vi "OF2 (SubVI).vi"() -> (0 "error out":errorcluster, 1 "Optical Flow Velocity X":T1, 2 "Optical Flow Previous Image":T1, 3 "Optical Flow Velocity Y":T1, 5 "Optical Flow Current Image":T1)   [LabVIEW 2014]
uses:
  <vilib>/vision/Image Controls.llb/IMAQ Image.ctl
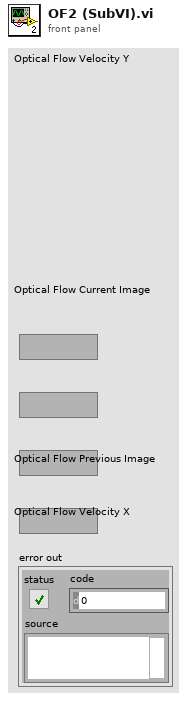
[diagram p1: front panel]
types:
  T1 = typedef "IMAQ Image.ctl" = refnum<image>
  T2 = typedef "Image Type" = u32
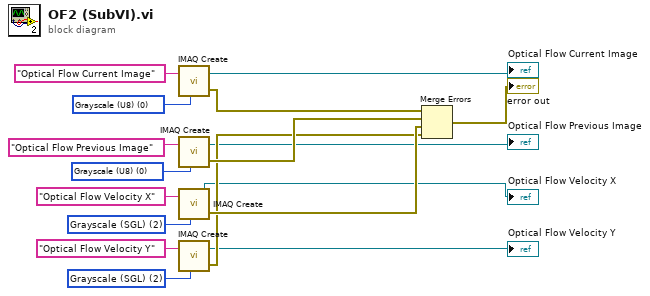
[diagram p0: block diagram]
diagram:
  w8 = T2 2 items=["Grayscale (U8)", "Grayscale (I16)", "Grayscale (SGL)", "Complex (CSG)", "RGB (U32)", "HSL (U32)", "RGB (U64)", "Grayscale (U16)"] ("Image Type")
  w7 = T2 0 items=["Grayscale (U8)", "Grayscale (I16)", "Grayscale (SGL)", "Complex (CSG)", "RGB (U32)", "HSL (U32)", "RGB (U64)", "Grayscale (U16)"] ("Image Type")
  w6 = T2 0 items=["Grayscale (U8)", "Grayscale (I16)", "Grayscale (SGL)", "Complex (CSG)", "RGB (U32)", "HSL (U32)", "RGB (U64)", "Grayscale (U16)"] ("Image Type")
  w5 = T2 2 items=["Grayscale (U8)", "Grayscale (I16)", "Grayscale (SGL)", "Complex (CSG)", "RGB (U32)", "HSL (U32)", "RGB (U64)", "Grayscale (U16)"] ("Image Type")
  n1 = call "IMAQ Create"("Image Name"="Optical Flow Current Image", "Image Type"=w6) -> ("New Image"=→"Optical Flow Current Image":T1, "error out"=w16:errorcluster)  [unwired: 2 in, 1 out]
  n2 = call "IMAQ Create"("Image Name"="Optical Flow Previous Image", "Image Type"=w7) -> ("New Image"=→"Optical Flow Previous Image":T1, "error out"=w15:errorcluster)  [unwired: 2 in, 1 out]
  n3 = call "IMAQ Create"("Image Name"="Optical Flow Velocity X", "Image Type"=w5) -> ("New Image"=→"Optical Flow Velocity X":T1, "error out"=w14:errorcluster)  [unwired: 2 in, 1 out]
  n4 = call "IMAQ Create"("Image Name"="Optical Flow Velocity Y", "Image Type"=w8) -> ("New Image"=→"Optical Flow Velocity Y":T1, "error out"=w13:errorcluster)  [unwired: 2 in, 1 out]
  n5 = Merge Errors(w16, w15, w14, w13) -> (→"error out":errorcluster)
